vi "TargetMet.vi"(0 "Target x (mm)":dbl, 5 "Target y (mm)":dbl, 7 "Current x (mm)":dbl, 9 "Current y (mm)":dbl, 11 "Dead Zone (mm)":dbl, 12 "error in (no error)":errorcluster) -> (4 "out":i32, 15 "error out":errorcluster)   [LabVIEW 2017, in "admittanceControllerLibrary.lvlib"]
doc: "This VI determines if the target has been reached.\n\nThe output is 1 if target reached.\n\nThe output is 0 if the target is not yet reached."
uses:
  admittanceControllerLibrary.lvlib
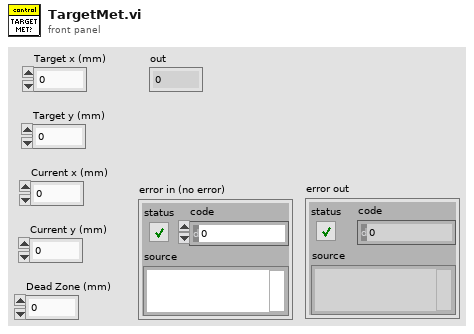
[diagram p1: front panel]
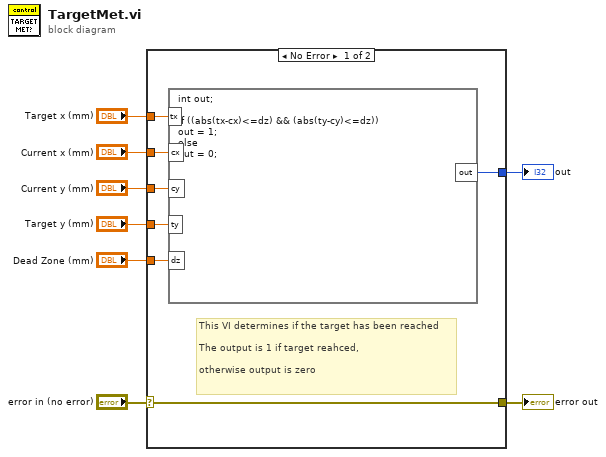
[diagram p0: block diagram]
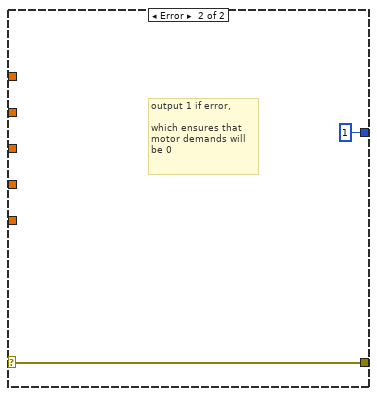
[diagram p2: hidden frame]
diagram:
  n1 = case shown="No Error" "error in (no error)" {
    selector: "error in (no error)" -> [w9 w17]
    tunnel: "Dead Zone (mm)" -> [w15 _]
    tunnel: "Target y (mm)" -> [w14 _]
    tunnel: "Current y (mm)" -> [w13 _]
    tunnel: "Current x (mm)" -> [w12 _]
    tunnel: "Target x (mm)" -> [w11 _]
    tunnel: [w10 1] -> w3
    tunnel: [w9 w17] -> w1
    frame No Error {
      # "This VI determines if the target has been reached\n\nThe output is 1 if target reahced,\n\notherwise output is zero"
      n2 = formula code="int out;\n\nif ((abs(tx-cx)<=dz) && (abs(ty-cy)<=dz))\nout = 1;\nelse \nout = 0;"("dz"=w15, "cx"=w12, "cy"=w13, "tx"=w11, "ty"=w14) -> ("out"=w10:i32)
    }
    frame Error {
      # "output 1 if error,\n\nwhich ensures that\nmotor demands will\nbe 0"
    }
  }
  "out" <- w3
  "error out" <- w1
